vi "InputHelper.vi"(3 "error in":errorcluster, 5 "Value":variant) -> (0 "error out":errorcluster, 1 "type":i32, 2 "Wafer ID":string)   [LabVIEW 2012, in "EpiWrapper.lvclass"]
uses:
  EpiWrapper.lvclass
  Controls/UserInput.ctl
  Controls/WaferSize.ctl
  Controls/MeasurementType.ctl
panel:
  out "WaferSize":i32
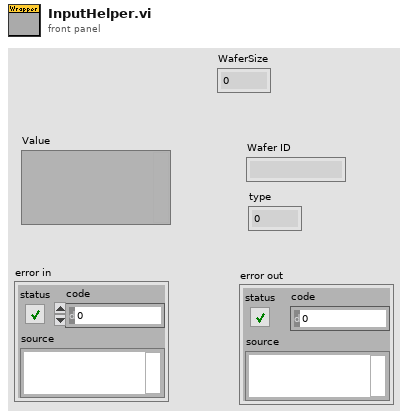
[diagram p1: front panel]
types:
  T1 = typedef "UserInput.ctl" = cluster{"Wafer ID":string, "Test Type":T2, "New":bool, "Save":bool, "Load":bool, "Cancel":bool, "Wafer Size":T3}
  T2 = typedef "MeasurementType.ctl" = enum16{"Initial", "Final"}
  T3 = typedef "WaferSize.ctl" = string
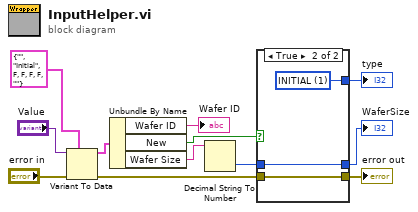
[diagram p0: block diagram]
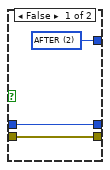
[diagram p2: hidden frame]
diagram:
  n1 = Variant To Data(error in="error in", type=T1 {"Wafer ID"="", "Test Type"=enum."Initial", "New"=FALSE, "Save"=FALSE, "Load"=FALSE, "Cancel"=FALSE, "Wafer Size"=""} ("Input"), Variant="Value") -> (data=w9:T1, error out=w4:errorcluster)
  n2 = Unbundle By Name(w9) -> ("Wafer ID"=→"Wafer ID":string, "New"=w10:bool, "Wafer Size"=w3:T3)
  n3 = Decimal String To Number(string=w3) -> (number=w1:i32)  [unwired: 2 in, 1 out]
  n4 = case shown="\"Initial\"" w10 {
    tunnel: [w15 w18] -> w11
    tunnel: [w14 w16] -> w5
    tunnel: w4 -> [w14 w16]
    tunnel: [w13 w17] -> w2
    tunnel: w1 -> [w13 w17]
    frame False {
      w15 = 2 items=["INITIAL"=1, "AFTER"=2] ("type")
    }
    frame True {
      w18 = 1 items=["INITIAL"=1, "AFTER"=2] ("type")
    }
  }
  "type" <- w11
  "error out" <- w5
  "WaferSize" <- w2
